vi "ProcessingRT.vi"(9 "SubstractedArray":dbl[](array[numeric]), 10 "Processing":u16, 11 "Array in":sgl[][](array[numeric])) -> (3 "Array out":sgl[][](array[numeric]))   [LabVIEW 2016]
uses:
  <vilib>/Analysis/baseanly.llb/Mean (DBL).vi
  <vilib>/Analysis/NI_AALBase.lvlib
  <vilib>/Analysis/NI_AALPro.lvlib
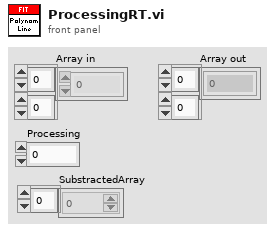
[diagram p1: front panel]
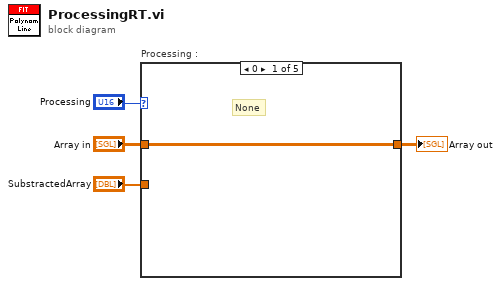
[diagram p0: block diagram]
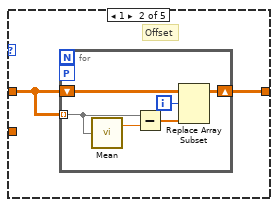
[diagram p2: hidden frame]
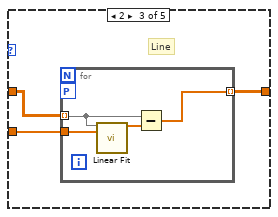
[diagram p3: hidden frame]
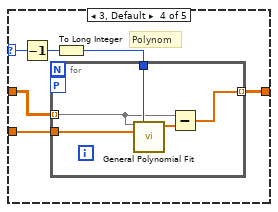
[diagram p4: hidden frame]
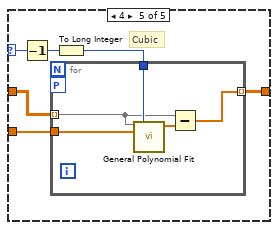
[diagram p5: hidden frame]
diagram:
  n1 = case "Processing :" shown="0" "Processing" {
    selector: "Processing" -> [_ _ _ w26 w37]
    tunnel: [w5 w7 w16 w21 w32] -> w1
    tunnel: "Array in" -> [w5 w6 w14 w23 w34]
    tunnel: "SubstractedArray" -> [_ _ w15 w22 w33]
    frame 0 {
      # "None"
    }
    frame 1 {
      # "Offset"
      n2 = for {
        tunnel: w6 -> [w13] mode=indexing
        shift-right: [w10] -> w7
        shift-left: w6 -> [w11]
        workers-P: _ -> [_]
        i -> [w9]
        n3 = call-poly <vilib>:"Mean.vi"("X"=w13) -> ("mean"=w12:dbl)  [unwired: 1 out]
        n4 = Subtract(x=w13, y=w12) -> (x-y=w8:dbl[])
        n5 = Replace Array Subset(array=w11, new element=w8, index (row)=w9) -> (w10:sgl[][])  [unwired: 1 in]
      }
    }
    frame 2 {
      # "Line"
      n6 = for {
        tunnel: w14 -> [w19] mode=indexing
        tunnel: w15 -> [w18]
        tunnel: [w17] -> w16 mode=indexing
        workers-P: _ -> [_]
        n7 = call <vilib>:"Linear Fit.vi"("Y"=w19, "X"=w18) -> ("Best Linear Fit"=w20:dbl[])  [unwired: 9 in, 4 out]
        n8 = Subtract(x=w19, y=w20) -> (x-y=w17:dbl[])
      }
    }
    frame 3, Default {
      # "Polynom"
      n9 = Decrement(x=w26) -> (x-1=w25:u16)
      n10 = To Long Integer(number=w25) -> (32bit integer=w24:i32)
      n11 = for {
        tunnel: w23 -> [w30] mode=indexing
        tunnel: w24 -> [w31]
        tunnel: w22 -> [w29]
        tunnel: [w27] -> w21 mode=indexing
        workers-P: _ -> [_]
        n12 = call <vilib>:"General Polynomial Fit.vi"("Y"=w30, "polynomial order"=w31, "X"=w29) -> ("Best Polynomial Fit"=w28:dbl[])  [unwired: 9 in, 3 out]
        n13 = Subtract(x=w30, y=w28) -> (x-y=w27:dbl[])
      }
    }
    frame 4 {
      # "Cubic"
      n14 = Decrement(x=w37) -> (x-1=w36:u16)
      n15 = To Long Integer(number=w36) -> (32bit integer=w35:i32)
      n16 = for {
        tunnel: w34 -> [w41] mode=indexing
        tunnel: w35 -> [w42]
        tunnel: w33 -> [w40]
        tunnel: [w38] -> w32 mode=indexing
        workers-P: _ -> [_]
        n17 = call <vilib>:"General Polynomial Fit.vi"("Y"=w41, "polynomial order"=w42, "X"=w40) -> ("Best Polynomial Fit"=w39:dbl[])  [unwired: 9 in, 3 out]
        n18 = Subtract(x=w41, y=w39) -> (x-y=w38:dbl[])
      }
    }
  }
  "Array out" <- w1
